vi "class_data.vi"() -> ()   [LabVIEW 2010, in "StimulatorAK101022TCP.lvclass"]
uses:
  StimulatorAK101022TCP.lvclass
  control_refs_cluster.ctl
panel:
  in  "control refs":T1
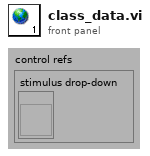
[diagram p1: front panel]
types:
  T1 = typedef "StimulatorAK101022TCP.lvclass/control_refs_cluster.ctl" = cluster{"stimulus drop-down":refnum<vi>}
diagram:
